vi "getXMLTestSuite.vi"(9 "indent level":i32, 10 "testsuite":T1={"name"="", "errors"=0, "skipped"=0, "tests"=0, "failures"=0, "time"=-1.0, "timestamp"=timestamp(0 s since 1904-01-01), "call-chain"=[], "properties"=variant}, 11 "Test Report in":refnum<class "Test Report.lvclass">) -> (1 "testsuite (end)":string="</testsuite>", 2 "testsuite (start)":string[](array[string]), 3 "Test Report":refnum<class "Test Report.lvclass">)   [LabVIEW 2013, in "Caraya.lvlib" / "Test Report.JUnit.lvclass"]
uses:
  Test Report.JUnit.lvclass
  testsuite -- cluster.ctl
  Test Report/Test Report.lvclass
  Test Report/Test Report.lvclass/Test Report.ctl
  MsgSerializer/MsgSerializer.lvclass/MsgSerializer.ctl
  MsgSerializer/MsgSerializer.lvclass
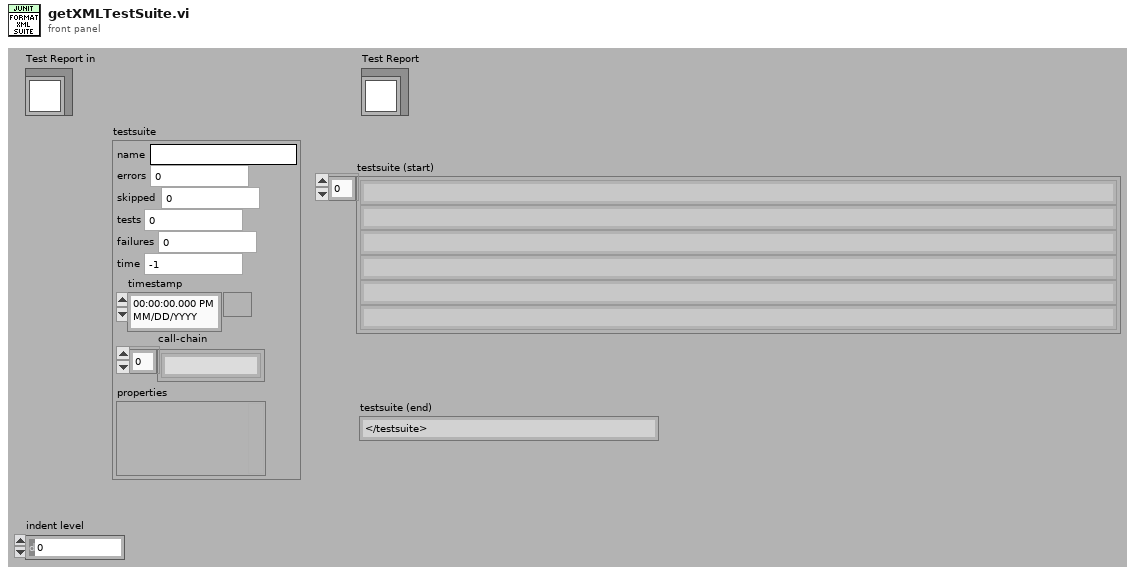
[diagram p1: front panel]
types:
  T1 = typedef "Caraya.lvlib/Test Report.JUnit.lvclass/testsuite -- cluster.ctl" = cluster{"name":string, "errors":u32, "skipped":u32, "tests":u32, "failures":u32, "time":dbl, "timestamp":timestamp, "call-chain":string[], "properties":variant}
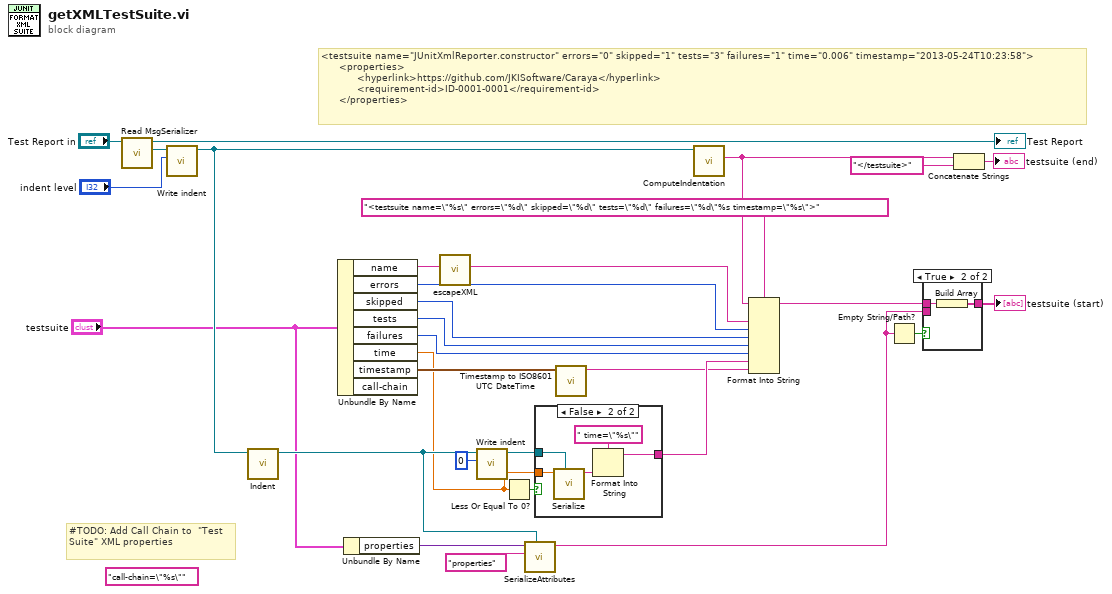
[diagram p0: block diagram]
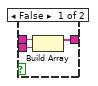
[diagram p3: hidden frame]
diagram:
  (unwired) "call-chain=\"%s\""
  # "#TODO: Add Call Chain to  \"Test Suite\" XML properties"
  # "<testsuite name=\"JUnitXmlReporter.constructor\" errors=\"0\" skipped=\"1\" tests=\"3\" failures=\"1\" time=\"0.006\" timestamp=\"2013-05-24T10:23:58\">\n      <properties>\n            <hyperlink>https://github.com/JKISoftware/Caraya</hyperlink>\n            <requirement-id>ID-0001-0001</requirement-id>\n      </properties>"
  n1 = call "Read MsgSerializer.vi"("Test Report in"="Test Report in") -> ("MsgSerializer"=w15:refnum<class "MsgSerializer.lvclass">, "Test Report out"=→"Test Report":refnum<class "Test Report.lvclass">)  [unwired: 9 in]
  n2 = call "Write indent.vi"("indent"="indent level", "MsgSerializer in"=w15) -> ("MsgSerializer out"=w4:refnum<class "MsgSerializer.lvclass">)  [unwired: 9 in]
  n3 = call "Indent.vi"("MsgSerializer in"=w4) -> ("MsgSerializer out"=w12:refnum<class "MsgSerializer.lvclass">)  [unwired: 10 in]
  n4 = Unbundle By Name("testsuite") -> ("name"=w24:string, "errors"=w30:u32, "skipped"=w29:u32, "tests"=w28:u32, "failures"=w27:u32, "time"=w11:dbl, "timestamp"=w26:timestamp)  [unwired: 1 out]
  n5 = Unbundle By Name("testsuite") -> ("properties"=w6:variant)
  n6 = call "escapeXML.vi"("Input String"=w24) -> ("XML-escaped String"=w23:string)  [unwired: 10 in]
  n7 = call "Write indent.vi"("indent"=0, "MsgSerializer in"=w12) -> ("MsgSerializer out"=w13:refnum<class "MsgSerializer.lvclass">)  [unwired: 9 in]
  n8 = Less Or Equal To 0?(x=w11) -> (x <= 0?=w10:bool)
  n9 = call "SerializeAttributes.vi"("MsgSerializer"=w12, "attribute name"="properties", "variant attribute"=w6) -> ("Serialized Message"=w18:string)  [unwired: 8 in]
  n10 = case shown="False" w10 {
    tunnel: [_ w34] -> w9
    tunnel: w11 -> [_ w33]
    tunnel: w13 -> [_ w31]
    frame True {
    }
    frame False {
      n11 = call-dynamic "Serialize.vi"("MsgSerializer"=w31, "Value"=w33) -> ("Serialized Message"=w32:string)  [unwired: 8 in, 1 out]
      n12 = Format Into String(format string=" time=\"%s\"", w32) -> (resulting string=w34:string)  [unwired: 2 in, 1 out]
    }
  }
  n13 = call <vilib>:"Timestamp to ISO8601 UTC DateTime.vi"("Timestamp (now)"=w26) -> ("ISO8601 UTC DateTime"=w7:string)  [unwired: 10 in]
  n14 = call "ComputeIndentation.vi"("MsgSerializer in"=w4) -> ("indentation"=w2:string)  [unwired: 10 in]
  n15 = Format Into String(format string="<testsuite name=\"%s\" errors=\"%d\" skipped=\"%d\" tests=\"%d\" failures=\"%d\"%s timestamp=\"%s\">", initial string=w2, w23, w30, w29, w28, w27, w9, w7) -> (resulting string=w1:string)  [unwired: 1 in, 1 out]
  n16 = Empty String/Path?(string/path=w18) -> (empty?=w19:bool)
  n17 = case shown="True" w19 {
    tunnel: [w38 w39] -> w17
    tunnel: w1 -> [w37 w40]
    tunnel: w18 -> [w36 _]
    frame False {
      n18 = Build Array(w37, w36) -> (w38:string[])
    }
    frame True {
      n19 = Build Array(w40) -> (w39:string[])
    }
  }
  "testsuite (start)" <- w17
  n20 = Concatenate Strings(w2, "</testsuite>" ("testsuite (end)")) -> (→"testsuite (end)":string)
